vi "Varian_PUMP_STATUS.vi"(8 "error in (no error)":errorcluster, 11 "VISA Refnum in":refnum<visa-resource-name>) -> (0 "error out":errorcluster, 1 "String":string, 2 "Numeric":dbl, 3 "VISA Refnum out":refnum<visa-resource-name>)   [LabVIEW 2015]
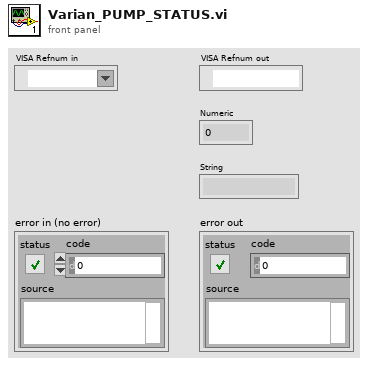
[diagram p1: front panel]
types:
  T1 = enum16{"START", "STOP", "REMOTE/SERIAL", "REMOTE", "SERIAL", "START/STOP", "PUMP STATUS", "Driving Frequency", "PUMP POWER", "PRESSURE"}
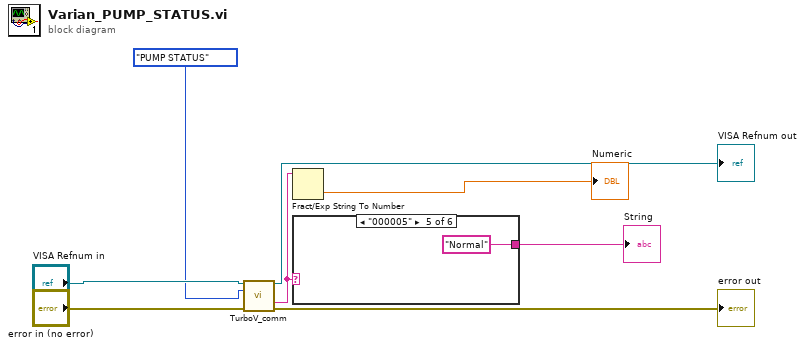
[diagram p0: block diagram]
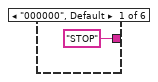
[diagram p2: hidden frame]
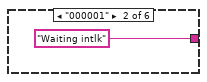
[diagram p3: hidden frame]
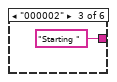
[diagram p4: hidden frame]
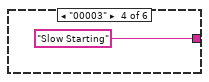
[diagram p5: hidden frame]
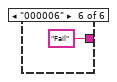
[diagram p6: hidden frame]
diagram:
  n1 = call "TurboV_comm.vi"("VISA resource name"="VISA Refnum in", "Command"=T1."PUMP STATUS", "error in (no error)"="error in (no error)") -> ("VISA resource name out"=→"VISA Refnum out":refnum<visa-resource-name>, "read buffer"=w4:string, "error out"=→"error out":errorcluster)  [unwired: 10 in]
  n2 = Fract/Exp String To Number(string=w4) -> (number=→"Numeric":dbl)  [unwired: 3 in, 1 out]
  n3 = case shown="\"000005\"" w4 {
    tunnel: ["STOP" "Waiting intlk" "Starting " "Slow Starting" "Normal" "Fail"] -> w8
    frame "000000", Default {
    }
    frame "000001" {
    }
    frame "000002" {
    }
    frame "00003" {
    }
    frame "000005" {
    }
    frame "000006" {
    }
  }
  "String" <- w8
